vi "Disconnect.vi"(8 "error in":errorcluster, 11 "Gen 2 in":refnum<class "Gen 2.lvclass">) -> (0 "error out":errorcluster, 3 "Gen 2 out":refnum<class "Gen 2.lvclass">)   [LabVIEW 2018, in "Gen 2.lvlib" / "Gen 2.lvclass"]
doc: "Close VISA resource session"
uses:
  Gen 2.lvclass
  PPLs/Laser/Parent/Laser.lvlibp/Laser.lvclass
  C:/Projects/LabVIEW/PPLs/Laser/Parent/Laser.lvlibp/Laser.lvclass
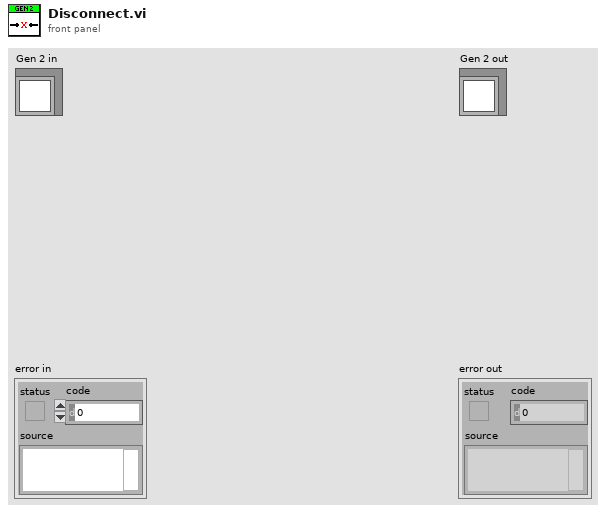
[diagram p1: front panel]
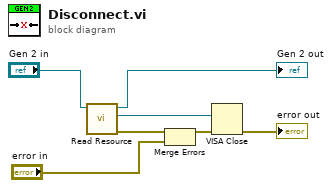
[diagram p0: block diagram]
diagram:
  n1 = call "Read Resource.vi"("Laser in"="Gen 2 in") -> ("error out"=w2:errorcluster, "Resource"=w6:refnum<visa-resource-name>, "Laser out"=→"Gen 2 out":refnum<class "Gen 2.lvclass">)  [unwired: 8 in]
  n2 = Merge Errors(w2, "error in") -> (w1:errorcluster)
  n3 = VISA Close(VISA resource name=w6, error in (no error)=w1) -> (error out=→"error out":errorcluster)
